vi "Piezo Message Loop.vi"(8 "error in (no error)":errorcluster, 10 "Data Notifiers":T1, 11 "Message Queues":T2) -> (0 "error out":errorcluster)   [LabVIEW 2013, in "Piezo.lvlib"]
uses:
  Piezo.lvlib
  support/Message Queue/All Message Queues.ctl
  support/Message Queue/Message Cluster.ctl
  support/Data Notifiers/All Data Notifiers.ctl
  Acquisition/APD Notifier Cluster.ctl
  Piezo display.ctl
  XY/XY Display.ctl
  Capacitive/Capacitive Signal Cluster.ctl
  Feedback/Error Signal.ctl
  Hardware Configuration.ctl
  Piezo State.ctl
  support/Message Queue/Enqueue Message (Single).vi
  <vilib>/Utility/error.llb/Error Cluster From Error Code.vi
  <vilib>/ErrorRing/Error Ring.xnode
  support/Message Queue/Message Queue.lvlib
  Acquisition/Acquisition.lvlib
  XY/XY.lvlib
  support/Data Notifiers/Data Notifiers.lvlib
  Capacitive/Capacitive.lvlib
  Feedback/Feedback.lvlib
panel:
  in  "MG17Piezo":refnum<k7>(container)
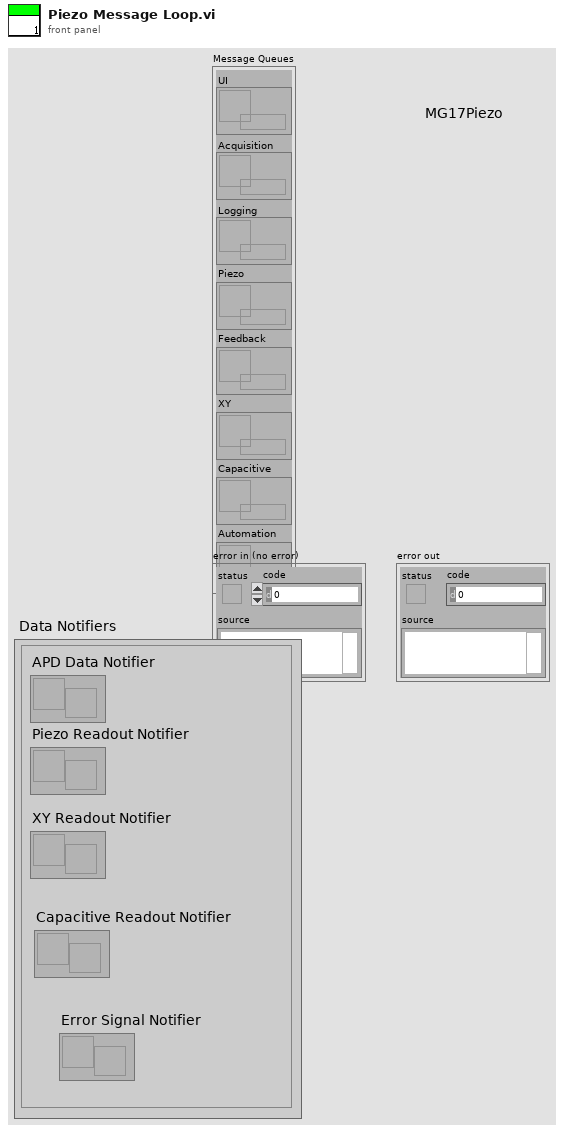
[diagram p1: front panel]
types:
  T1 = typedef "Data Notifiers.lvlib/All Data Notifiers.ctl" = cluster{"APD Data Notifier":refnum<notifier>, "Piezo Readout Notifier":refnum<notifier>, "XY Readout Notifier":refnum<notifier>, "Capacitive Readout Notifier":refnum<notifier>, "Error Signal Notifier":refnum<notifier>}
  T2 = typedef "Message Queue.lvlib/All Message Queues.ctl" = cluster{"UI":refnum<queue>, "Acquisition":refnum<queue>, "Logging":refnum<queue>, "Piezo":refnum<queue>, "Feedback":refnum<queue>, "XY":refnum<queue>, "Capacitive":refnum<queue>, "Automation":refnum<queue>}
  T3 = typedef "Piezo.lvlib/Hardware Configuration.ctl" = cluster{"Piezo Serial Number":i32, "MG17Piezo":refnum<k7>, "Setpoint (um)":sgl}
  T4 = typedef "Piezo.lvlib/Piezo State.ctl" = enum16{"Idle", "Acquiring"}
  T5 = typedef "Acquisition.lvlib/APD Notifier Cluster.ctl" = cluster{"data":dbl[][], "t0":i32}
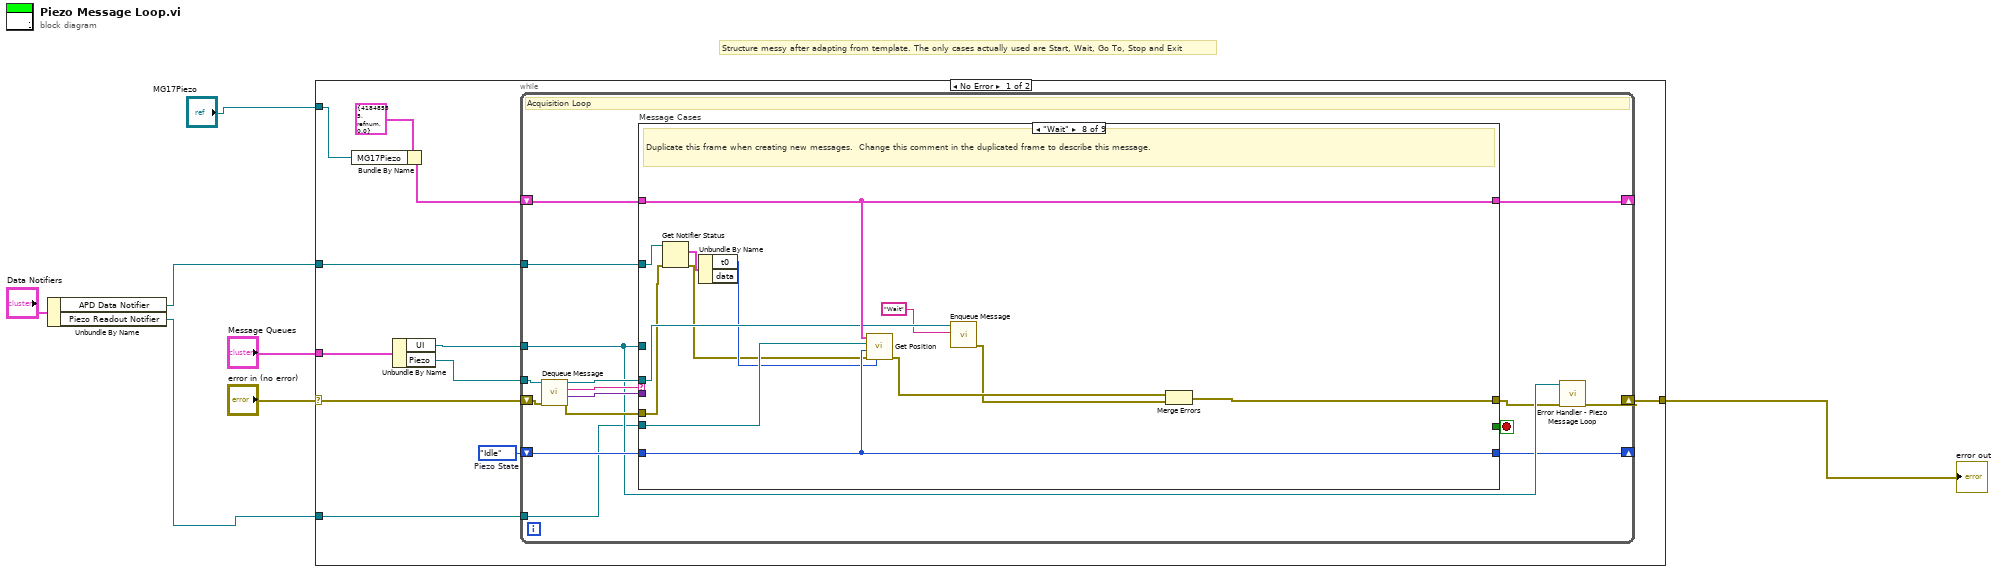
[diagram p0: block diagram]
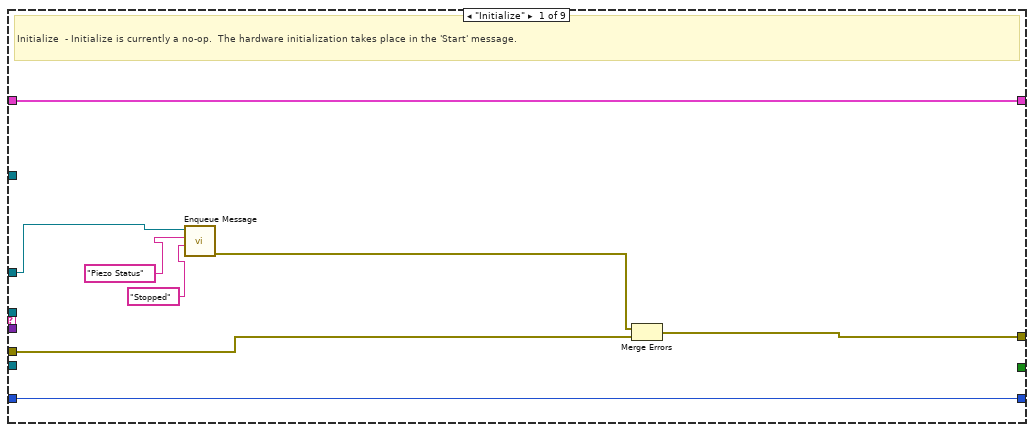
[diagram p2: hidden frame]
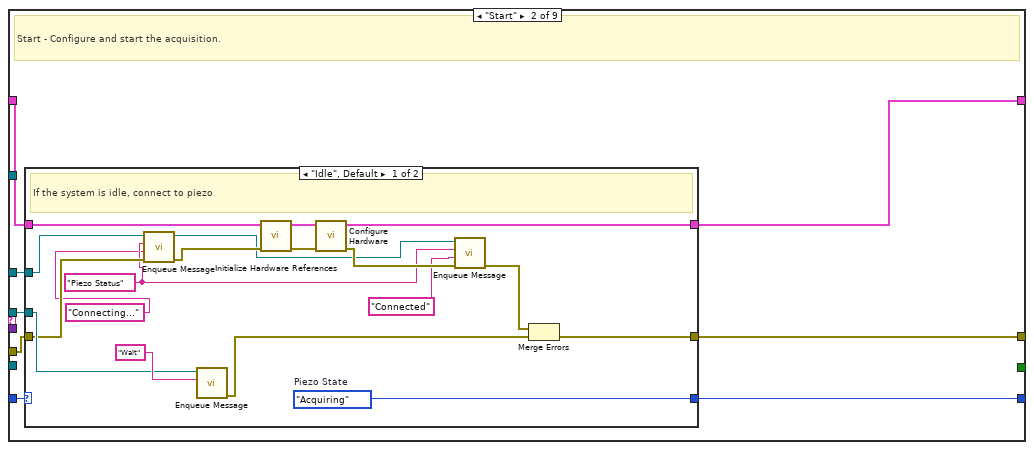
[diagram p3: hidden frame]
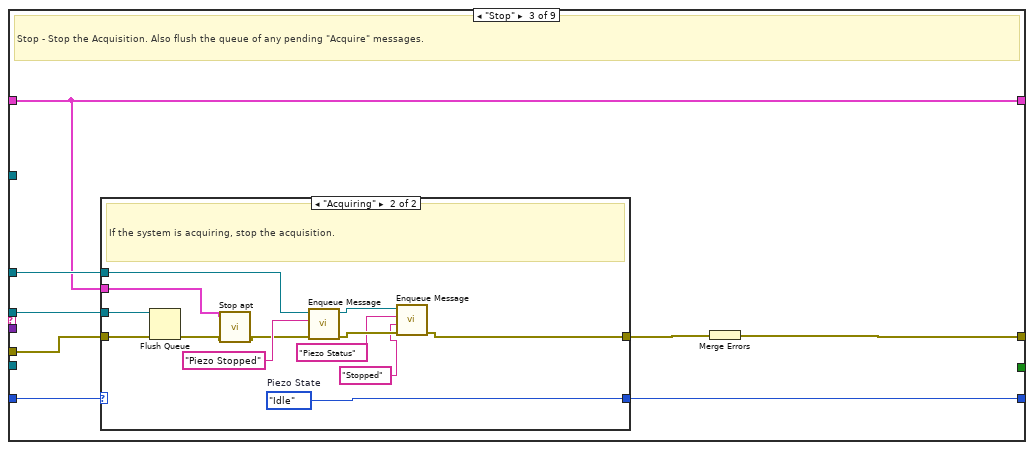
[diagram p5: hidden frame]
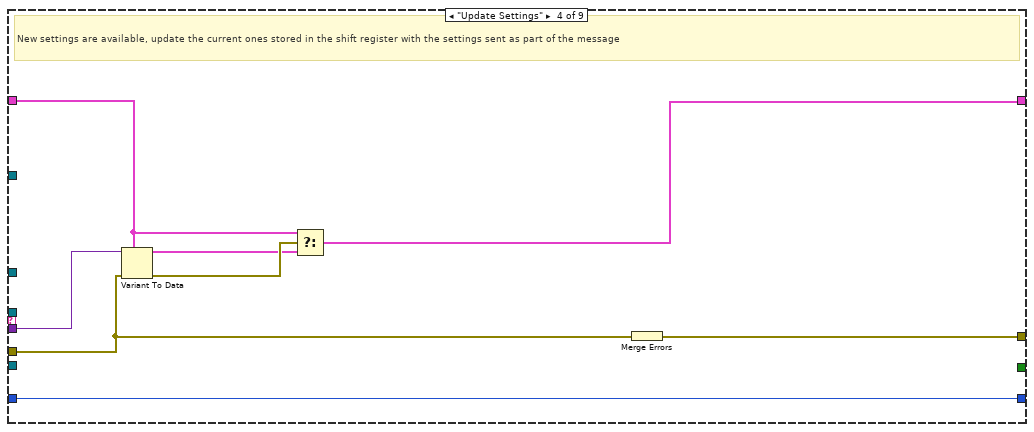
[diagram p7: hidden frame]
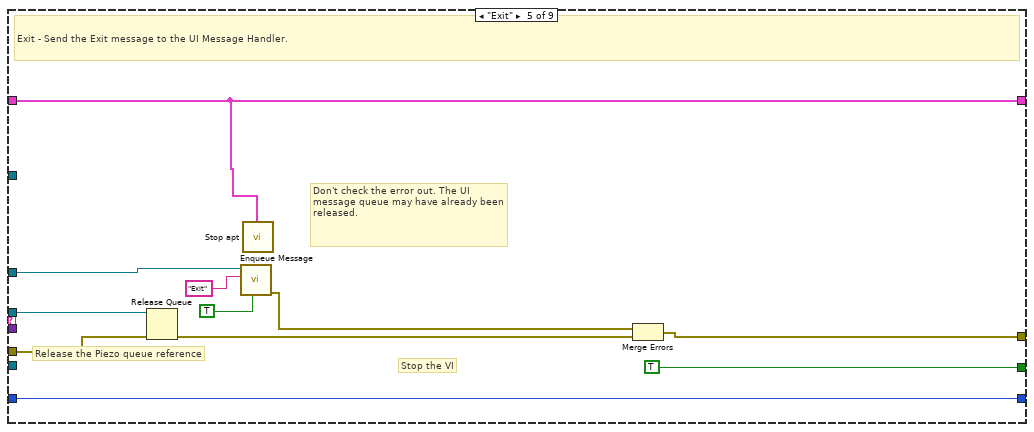
[diagram p8: hidden frame]
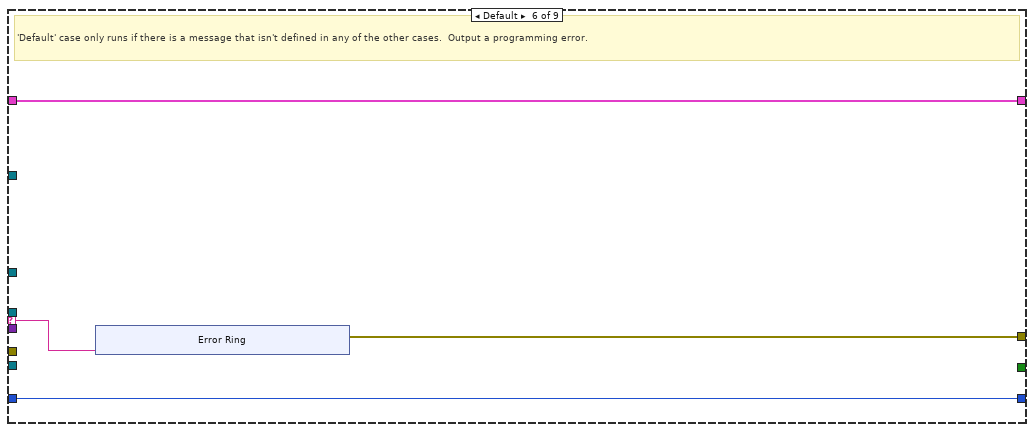
[diagram p9: hidden frame]
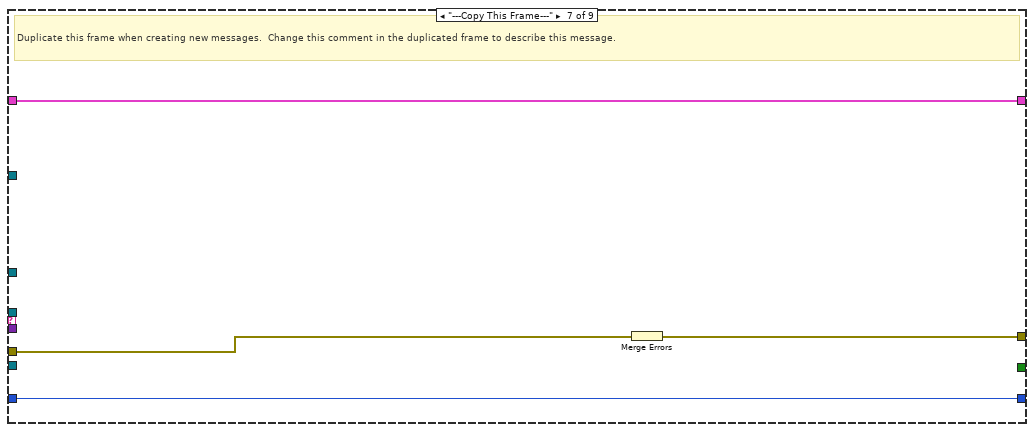
[diagram p10: hidden frame]
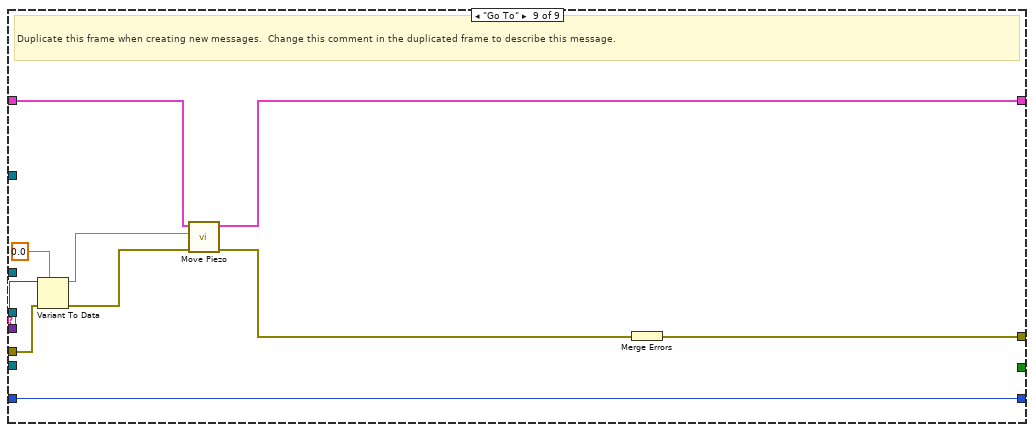
[diagram p11: hidden frame]
diagram:
  # "Structure messy after adapting from template. The only cases actually used are Start, Wait, Go To, Stop and Exit"
  n1 = Unbundle By Name("Data Notifiers") -> ("APD Data Notifier"=w2:refnum<notifier>, "Piezo Readout Notifier"=w1:refnum<notifier>)
  n2 = case shown="No Error" "error in (no error)" {
    selector: "error in (no error)" -> [w10 w152]
    tunnel: "Message Queues" -> [w18 _]
    tunnel: [w16 w152] -> w6
    tunnel: "MG17Piezo" -> [w11 _]
    tunnel: w1 -> [w9 _]
    tunnel: w2 -> [w8 _]
    frame No Error {
      w12 = Piezo_State."Idle"  # Piezo State
      n3 = Bundle By Name(cluster=T3 {"Piezo Serial Number"=41848555, "MG17Piezo"=refnum, "Setpoint (um)"=0.0} ("Hardware Configuration"), "MG17Piezo"=w11) -> (w14:T3)
      n4 = Unbundle By Name(w18) -> ("UI"=w15:refnum<queue>, "Piezo"=w17:refnum<queue>)
      n5 = while {
        tunnel: w17 -> [w27]
        shift-right: [w22] -> _
        shift-left: w14 -> [w34]
        shift-right: [w24] -> w16
        shift-left: w10 -> [w32]
        tunnel: w15 -> [w25]
        shift-right: [w23] -> _
        shift-left: w12 -> [w26]
        tunnel: w9 -> [w20]
        tunnel: w8 -> [w19]
        stop <- w33 stop-if-true
        # "Acquisition Loop"
        n6 = call "Dequeue Message.vi"("error in (no error)"=w32, "Message Queue"=w27) -> ("error out"=w31:errorcluster, "Message Data"=w29:variant, "Message"=w30:string, "dup Message Queue"=w28:refnum<queue>)  [unwired: 6 in]
        n7 = case "Message Cases" shown="\"Wait\"" w30 {
          selector: w30 -> [_ _ _ _ _ w117 _ _ _]
          tunnel: w28 -> [_ w47 w77 _ w109 _ _ w136 _]
          tunnel: w31 -> [w41 w48 w78 w97 w111 _ w128 w131 w143]
          tunnel: [w42 w50 w79 w102 w112 w116 w127 w141 w151] -> w21
          tunnel: w34 -> [w39 w49 w72 w98 w107 w114 w125 w137 w149]
          tunnel: [_ _ _ _ TRUE _ _ _ _] -> w33
          tunnel: w29 -> [_ _ _ w101 _ _ _ _ w146]
          tunnel: w25 -> [w37 w43 w76 _ w104 _ _ _ _]
          tunnel: w26 -> [w40 w46 w75 w96 w108 w115 w126 w139 w150]
          tunnel: [w40 w45 w74 w96 w108 w115 w126 w139 w150] -> w23
          tunnel: [w39 w44 w72 w95 w107 w114 w125 w137 w148] -> w22
          tunnel: w20 -> [_ _ _ _ _ _ _ w138 _]
          tunnel: w19 -> [_ _ _ _ _ _ _ w130 _]
          frame "Initialize" {
            # "Initialize  - Initialize is currently a no-op.  The hardware initialization takes place in the 'Start' message."
            n8 = call-poly "Enqueue Message.vi"("Message Data"="Stopped" ("Message"), "Message"="Piezo Status", "Message Queue"=w37) -> ("error out"=w36:errorcluster)  [unwired: 7 in, 1 out]
            n9 = Merge Errors(w36, w41) -> (w42:errorcluster)
          }
          frame "Start" {
            # "Start - Configure and start the acquisition."
            n10 = case shown="\"Idle\", Default" w46 {
              selector: w46 -> [_ w69]
              tunnel: [w68 w71] -> w50
              tunnel: w49 -> [w67 w70]
              tunnel: w48 -> [w55 w71]
              tunnel: w47 -> [w61 _]
              tunnel: [w64 w70] -> w44
              tunnel: [w63 w69] -> w45
              tunnel: w43 -> [w56 _]
              frame "Idle", Default {
                w52 = "Piezo Status" ("Message")
                w63 = Piezo_State."Acquiring"  # Piezo State
                # "If the system is idle, connect to piezo"
                n11 = call-poly "Enqueue Message.vi"("error in (no error)"=w55, "Message Data"="Connecting..." ("Message"), "Message"=w52, "Message Queue"=w56) -> ("error out"=w54:errorcluster, "dup Message Queue"=w53:refnum<queue>)  [unwired: 6 in]
                n12 = call-poly "Enqueue Message.vi"("Message"="Wait", "Message Queue"=w61) -> ("error out"=w60:errorcluster)  [unwired: 8 in, 1 out]
                n13 = call "Initialize Hardware References.vi"("error in (no error)"=w54, "Hardware Resources In"=w67) -> ("error out"=w66:errorcluster, "Hardware Resources Out"=w65:T3)  [unwired: 8 in]
                n14 = call "Configure Hardware.vi"("error in (no error)"=w66, "Hardware Resources In"=w65) -> ("error out"=w59:errorcluster, "Hardware Resources Out"=w64:T3)  [unwired: 8 in]
                n15 = call-poly "Enqueue Message.vi"("error in (no error)"=w59, "Message Data"="Connected" ("Message"), "Message"=w52, "Message Queue"=w53) -> ("error out"=w58:errorcluster)  [unwired: 6 in, 1 out]
                n16 = Merge Errors(w58, w60) -> (w68:errorcluster)
              }
              frame "Acquiring" {
                # "The system is already acquiring. Ignore the \"Start\" message."
              }
            }
          }
          frame "Stop" {
            # "Stop - Stop the Acquisition. Also flush the queue of any pending \"Acquire\" messages."
            n17 = case shown="\"Acquiring\"" w75 {
              selector: w75 -> [w81 _]
              tunnel: w78 -> [w80 w94]
              tunnel: w72 -> [_ w90]
              tunnel: w77 -> [_ w93]
              tunnel: w76 -> [_ w92]
              tunnel: [w81 w87] -> w74
              tunnel: [w80 w84] -> w73
              frame "Idle", Default {
                # "The system is already idle. Ignore the \"Stop\" message."
              }
              frame "Acquiring" {
                w87 = Piezo_State."Idle"  # Piezo State
                # "If the system is acquiring, stop the acquisition."
                n18 = Flush Queue(queue=w93, error in (no error)=w94) -> (error out=w89:errorcluster)  [unwired: 2 out]
                n19 = call "Stop apt.vi"("error in (no error)"=w89, "Hardware Resources In"=w90) -> ("error out"=w88:errorcluster)  [unwired: 9 in]
                n20 = call-poly "Enqueue Message.vi"("error in (no error)"=w88, "Message"="Piezo Stopped", "Message Queue"=w92) -> ("error out"=w85:errorcluster, "dup Message Queue"=w86:refnum<queue>)  [unwired: 7 in]
                n21 = call-poly "Enqueue Message.vi"("error in (no error)"=w85, "Message Data"="Stopped" ("Message"), "Message"="Piezo Status", "Message Queue"=w86) -> ("error out"=w84:errorcluster)  [unwired: 6 in, 1 out]
              }
            }
            n22 = Merge Errors(w73) -> (w79:errorcluster)
          }
          frame "Update Settings" {
            # "New settings are available, update the current ones stored in the shift register with the settings sent as part of the message"
            n23 = Variant To Data(error in=w97, type=w98, Variant=w101) -> (data=w99:T3, error out=w100:errorcluster)
            n24 = Select(t=w98, s=w100, f=w99) -> (s? t:f=w95:T3)
            n25 = Merge Errors(w97) -> (w102:errorcluster)
          }
          frame "Exit" {
            # "Don't check the error out. The UI message queue may have already been released."
            # "Release the Piezo queue reference"
            # "Stop the VI"
            # "Exit - Send the Exit message to the UI Message Handler."
            n26 = Release Queue(queue=w109, error in (no error)=w111) -> (error out=w110:errorcluster)  [unwired: 1 in, 2 out]
            n27 = call-poly "Enqueue Message.vi"("Priority Message? (F)"=TRUE, "Message"="Exit", "Message Queue"=w104) -> ("error out"=w103:errorcluster)  [unwired: 7 in, 1 out]
            n28 = call "Stop apt.vi"("Hardware Resources In"=w107) -> ()  [unwired: 10 in, 1 out]
            n29 = Merge Errors(w103, w110) -> (w112:errorcluster)
          }
          frame Default {
            # "'Default' case only runs if there is a message that isn't defined in any of the other cases.  Output a programming error."
            n30 = xnode "Error Ring"("parameter 0"=w117) -> ("error out"=w116:errorcluster)
          }
          frame "---Copy This Frame---" {
            # "Duplicate this frame when creating new messages.  Change this comment in the duplicated frame to describe this message."
            n31 = Merge Errors(w128) -> (w127:errorcluster)
          }
          frame "Wait" {
            # "Duplicate this frame when creating new messages.  Change this comment in the duplicated frame to describe this message."
            n32 = Get Notifier Status(notifier=w130, error in (no error)=w131) -> (current notification=w129:T5, error out=w132:errorcluster)  [unwired: 3 out]
            n33 = Unbundle By Name(w129) -> ("t0"=w133:i32)  [unwired: 1 out]
            n34 = call "Get Position.vi"("Counter Time"=w133, "error in (no error)"=w132, "Piezo State"=w139, "notifier out"=w138, "Hardware Resources In"=w137) -> ("error out"=w140:errorcluster)  [unwired: 5 in, 1 out]
            n35 = call-poly "Enqueue Message.vi"("Message"="Wait", "Message Queue"=w136) -> ("error out"=w134:errorcluster)  [unwired: 8 in, 1 out]
            n36 = Merge Errors(w140, w134) -> (w141:errorcluster)
          }
          frame "Go To" {
            # "Duplicate this frame when creating new messages.  Change this comment in the duplicated frame to describe this message."
            n37 = Variant To Data(error in=w143, type=sgl 0.0, Variant=w146) -> (data=w145:sgl, error out=w142:errorcluster)
            n38 = call "Move Piezo.vi"("error in (no error)"=w142, "Move to (um)"=w145, "Hardware Resources In"=w149) -> ("error out"=w147:errorcluster, "Hardware Resources Out"=w148:T3)  [unwired: 7 in]
            n39 = Merge Errors(w147) -> (w151:errorcluster)
          }
        }
        n40 = call "Error Handler - Piezo Message Loop.vi"("error in (no error)"=w21, "Message Queue"=w25) -> ("dup error in"=w24:errorcluster)  [unwired: 8 in, 1 out]
      }
    }
    frame Error {
    }
  }
  "error out" <- w6
